vi "Set XRT-U Angle.vi"(8 "error in (no error)":errorcluster, 10 "Angle (°)":dbl, 11 "Inst.Xeryon-Rotator in":refnum<class "Inst.Xeryon-Rotator.lvclass">) -> (0 "error out":errorcluster, 3 "Inst.Xeryon-Rotator out":refnum<class "Inst.Xeryon-Rotator.lvclass">)   [LabVIEW 2019, in "Inst.Xeryon-Rotator.lvclass"]
uses:
  <userlib>/LevyLab/Xeryon-Rotator/lvsrc/SMOs/Inst.Xeryon-Rotator/Inst.Xeryon-Rotator.lvclass
  <userlib>/LevyLab/Xeryon-Rotator/lvsrc/SMOs/Inst.Xeryon-Rotator/Inst.Xeryon-Rotator.lvclass/Inst.Xeryon-Rotator.ctl
  <userlib>/LevyLab/Xeryon-Rotator/lvsrc/drivers/Class/Controller/Controller.lvclass
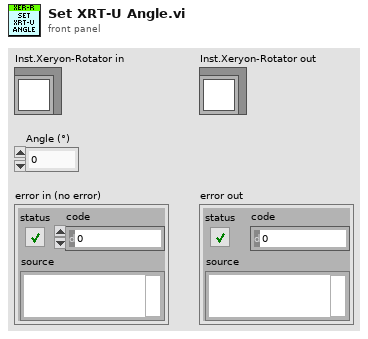
[diagram p1: front panel]
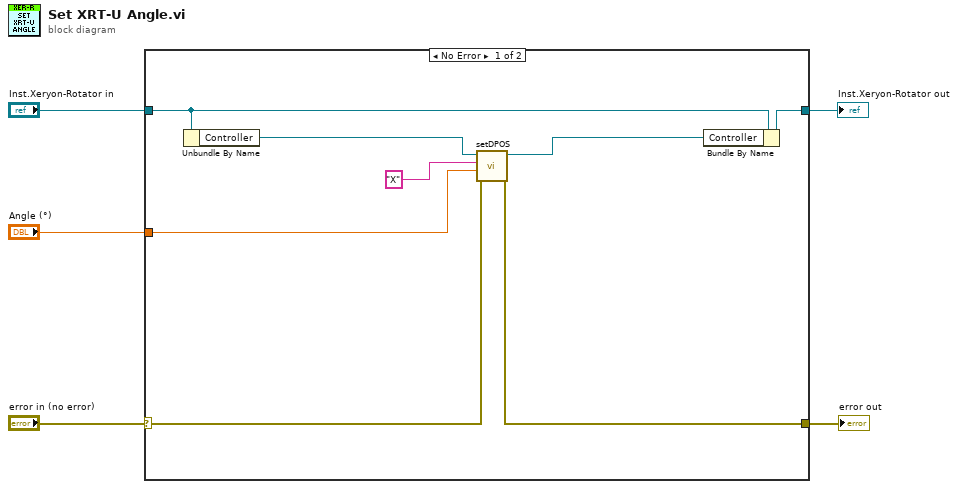
[diagram p0: block diagram]
diagram:
  n1 = case shown="No Error" "error in (no error)" {
    selector: "error in (no error)" -> [w7 w15]
    tunnel: [w13 w14] -> w5
    tunnel: "Inst.Xeryon-Rotator in" -> [w12 w14]
    tunnel: "Angle (°)" -> [w9 _]
    tunnel: [w6 w15] -> w1
    frame No Error {
      n2 = Unbundle By Name(w12) -> ("Controller"=w10:refnum<class "Controller.lvclass">)
      n3 = call-dynamic "setDPOS.vi"("error in (no error)"=w7, "DPOS In Current Units"=w9, "Axis Letter"="X", "Controller in"=w10) -> ("error out"=w6:errorcluster, "Controller out"=w11:refnum<class "Controller.lvclass">)  [unwired: 6 in]
      n4 = Bundle By Name(cluster=w12, "Controller"=w11) -> (w13:refnum<class "Inst.Xeryon-Rotator.lvclass">)
    }
    frame Error {
    }
  }
  "error out" <- w1
  "Inst.Xeryon-Rotator out" <- w5
